vi "Read.vi"(8 "error in (no error)":errorcluster, 9 "Variant":variant, 11 "VISA in":refnum<class "VISA.lvclass">) -> (0 "error out":errorcluster, 2 "String":string, 3 "VISA out":refnum<class "VISA.lvclass">)   [LabVIEW 2013, in "Protocol Classes.lvlib" / "VISA.lvclass"]
uses:
  VISA.lvclass
  Protocol Parent/Methods/Read Parameter.ctl
  VISA.lvclass/VISA.ctl
  Read Ref.vi
  Write Ref.vi
  Protocol Parent/Protocol Parent.lvclass
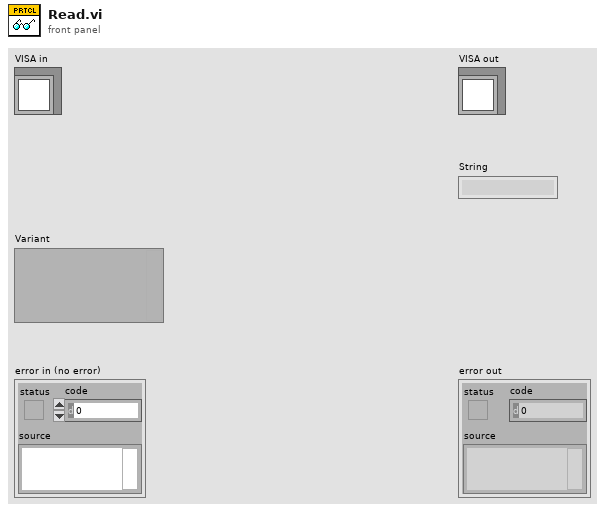
[diagram p1: front panel]
types:
  T1 = typedef "Protocol Classes.lvlib/Protocol Parent.lvclass/Read Parameter.ctl" = cluster{"Wait Type":enum16{"Byte Count", "Wait sec"}, "Wait Value":dbl}
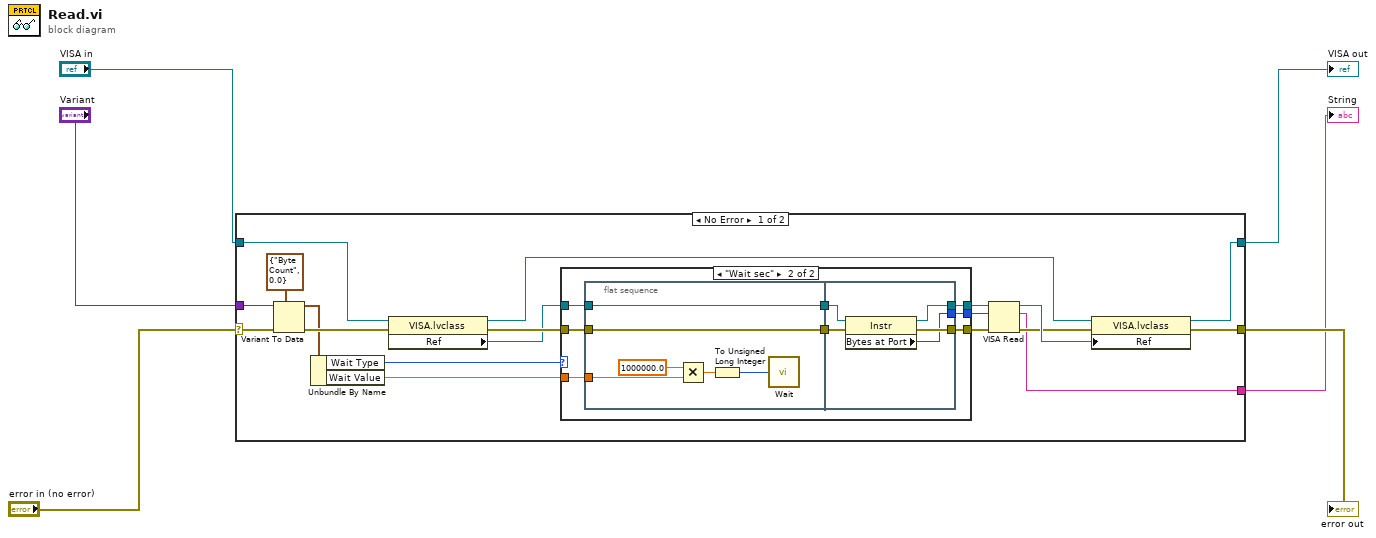
[diagram p0: block diagram]
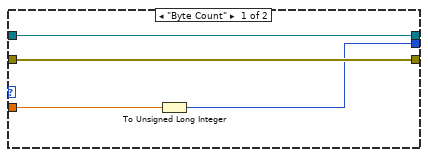
[diagram p2: hidden frame]
diagram:
  n1 = case shown="No Error" "error in (no error)" {
    selector: "error in (no error)" -> [w19 w50]
    tunnel: "VISA in" -> [w25 w49]
    tunnel: [w22 w50] -> w3
    tunnel: [w20 w49] -> w1
    tunnel: "Variant" -> [w17 _]
    tunnel: [w8 _] -> w2
    frame No Error {
      n2 = Variant To Data(error in=w19, type=T1 {"Wait Type"=enum."Byte Count", "Wait Value"=0.0} ("Read Parameter"), Variant=w17) -> (data=w16:T1, error out=w18:errorcluster)
      n3 = Unbundle By Name(w16) -> ("Wait Type"=w10:enum16{"Byte Count", "Wait sec"}, "Wait Value"=w9:dbl)
      n4 = property class="VISA.lvclass"(reference=w25, error in=w18) -> (reference out=w21:refnum<class "VISA.lvclass">, error out=w15:errorcluster, "Ref"=w14:refnum<visa-resource-name>)
      n5 = case shown="\"Wait sec\"" w10 {
        tunnel: w15 -> [w29 w37]
        tunnel: w14 -> [w28 w36]
        tunnel: [w29 w35] -> w13
        tunnel: [w28 w34] -> w12
        tunnel: [w26 w33] -> w11
        tunnel: w9 -> [w27 w30]
        frame "Byte Count" {
          n6 = To Unsigned Long Integer(number=w27) -> (unsigned 32bit integer=w26:u32)
        }
        frame "Wait sec" {
          n7 = flat-sequence {
            tunnel: w36 -> [w42]
            tunnel: w37 -> [w43]
            tunnel: [w43] -> w32
            tunnel: [w42] -> w31
            tunnel: w30 -> [w39]
            tunnel: [w46] -> w35
            tunnel: [w45] -> w34
            tunnel: [w44] -> w33
            tunnel: w32 -> [w48]
            tunnel: w31 -> [w47]
            frame #0 {
              n8 = Multiply(x=1000000.0, y=w39) -> (x*y=w41:dbl)
              n9 = To Unsigned Long Integer(number=w41) -> (unsigned 32bit integer=w38:u32)
              n10 = call "Wait"("Count(uSec)"=w38) -> ()  [unwired: 1 out]
            }
            frame #1 {
              n11 = property class="Instr"(reference=w47, error in=w48) -> (reference out=w45:refnum<visa-resource-name>, error out=w46:errorcluster, "Bytes at Port"=w44:u32)
            }
          }
        }
      }
      n12 = VISA Read(VISA resource name=w12, byte count=w11, error in (no error)=w13) -> (VISA resource name out=w24:refnum<visa-resource-name>, read buffer=w8:string, error out=w23:errorcluster)  [unwired: 1 out]
      n13 = property class="VISA.lvclass"(reference=w21, error in=w23, "Ref"=w24) -> (reference out=w20:refnum<class "VISA.lvclass">, error out=w22:errorcluster)
    }
    frame Error {
    }
  }
  "error out" <- w3
  "VISA out" <- w1
  "String" <- w2
